vi "Postion_PWM.vi"(1 "Position_KD":dbl, 2 "Position_KP":dbl, 3 "Encoder":dbl) -> (0 "Postion_PWM":dbl)   [LabVIEW 2018]
uses:
  Global_variables.vi
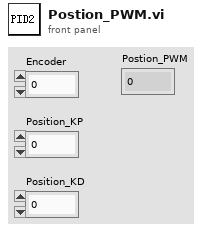
[diagram p1: front panel]
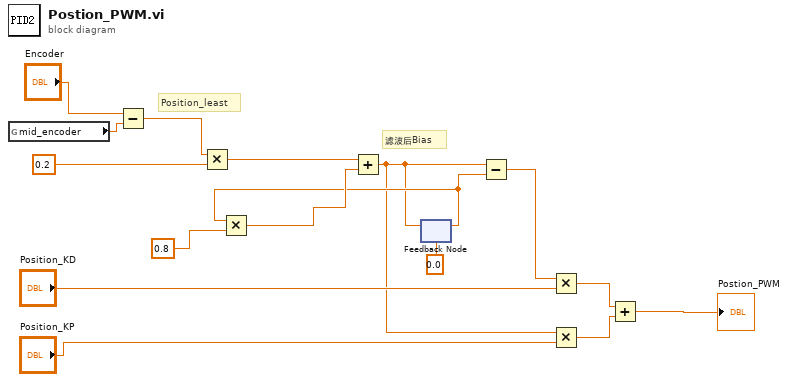
[diagram p0: block diagram]
diagram:
  # "滤波后Bias"
  # "Position_least"
  n1 = global read "Global_variables.vi" "mid_encoder"() -> (w1:dbl)
  n2 = Subtract(x="Encoder", y=w1) -> (x-y=w15:dbl)
  n3 = Multiply(x=w15, y=0.2) -> (x*y=w12:dbl)
  n4 = feedback #1(0.0) -> (w3:dbl)
  n5 = Multiply(x=w3, y=0.8) -> (x*y=w11:dbl)
  n6 = Add(x=w12, y=w11) -> (x+y=w2:dbl)
  n7 = feedback-in #1(w2) -> ()
  n8 = Subtract(x=w2, y=w3) -> (x-y=w9:dbl)
  n9 = Multiply(x=w9, y="Position_KD") -> (x*y=w6:dbl)
  n10 = Multiply(x=w2, y="Position_KP") -> (x*y=w5:dbl)
  n11 = Add(x=w6, y=w5) -> (x+y=→"Postion_PWM":dbl)
